vi "Build Monitor Cluster.vi"(8 "error in":errorcluster, 11 "custom device ref in":T4=18446744073709551615 format="%.0x") -> (0 "error out":errorcluster, 2 "Monitor cluster out":T1={"channel #"=0, "channel handle"=0, "InstrumentHandle_board"=0, "InstrumentHandle_port"=0, "Queue ID"=0, "channel settings"={"Monitor Settings"={"DefaultCronoMode"=0, "GlbMonBufferSizeIn"=0, "CaptureMode"=0, "MaxFileSize MB (1)"=1, "Strobe"=0, "TriggerPosition"=0}, "Rx Board"=0, "Rx Port"=0}, "File Reference"=refnum, "Monitor Log Directory"=""} {"channel settings"."Monitor Settings"."Strobe" items=["FDX_MON_STROBE_DIS", "FDX_MON_STROBE_STOP", "FDX_MON_STROBE_START"]; "channel settings"."Monitor Settings"."CaptureMode" items=["FDX_MON_SINGLE ", "FDX_MON_CONTINUOUS", "FDX_MON_SELECTIVE", "FDX_MON_RECORDING", "FDX_MON_REROS", "FDX_MON_HMU"]; "channel settings"."Monitor Settings"."DefaultCronoMode" items=["FDX_RX_DEFAULT_ENA_CNT", "FDX_RX_DEFAULT_MON_ENA_ALL", "FDX_RX_DEFAULT_MON_ENA_GOOD"]}, 3 "custom device ref out":T4 format="%.0x")   [LabVIEW 2020, in "afdx_custom_device Scripting.lvlib"]
uses:
  afdx_custom_device Scripting.lvlib
  <vilib>/NI VeriStand/Custom Device API/Custom Device Item Ref.ctl
  Engine/Implementation/Monitor Execution Unit/hardware_channels_rx.ctl
  Engine/Implementation/Monitor Execution Unit/channel_settings_rx.ctl
  AIM LabVIEW src/src/_controls/session_monitor_config.ctl
  Constants.vi
  <vilib>/NI VeriStand/Custom Device API/Get Item Property (U32).vi
  <vilib>/NI VeriStand/Custom Device API/Custom Device API.lvlib
  AIM LabVIEW src/src/AIM664LV.lvlib
  Engine/Implementation/Monitor Execution Unit/Monitor Execution Unit.lvclass
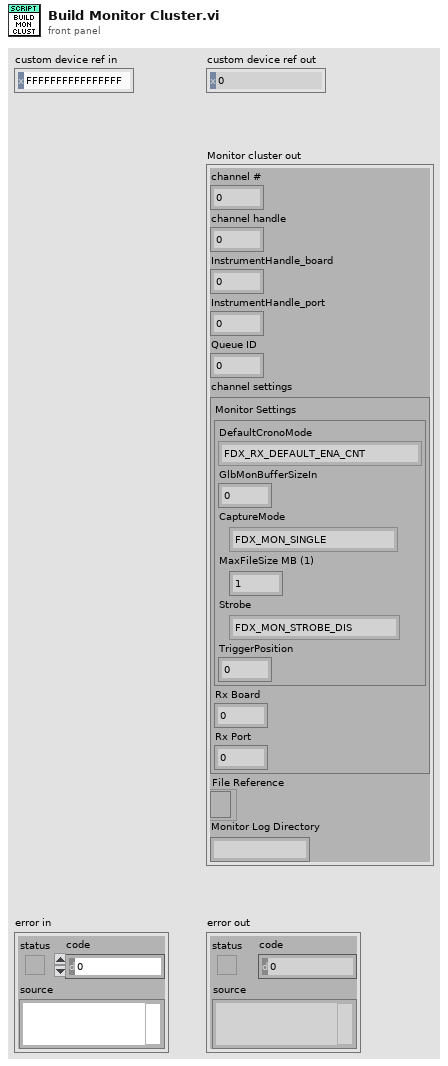
[diagram p1: front panel]
types:
  T1 = typedef "afdx_custom_device Engine.lvlib/Implementation.lvlib/Monitor Execution Unit.lvclass/hardware_channels_rx.ctl" = cluster{"channel #":u16, "channel handle":u64, "InstrumentHandle_board":u32, "InstrumentHandle_port":u32, "Queue ID":u32, "channel settings":T2, "File Reference":refnum<file>, "Monitor Log Directory":string}
  T2 = typedef "afdx_custom_device Engine.lvlib/Implementation.lvlib/Monitor Execution Unit.lvclass/channel_settings_rx.ctl" = cluster{"Monitor Settings":T3, "Rx Board":u32, "Rx Port":u32}
  T3 = typedef "AIM664LV.lvlib/session_monitor_config.ctl" = cluster{"DefaultCronoMode":u32, "GlbMonBufferSizeIn":u32, "CaptureMode":u32, "MaxFileSize MB (1)":u32, "Strobe":u32, "TriggerPosition":u32}
  T4 = typedef "Custom Device API.lvlib/Custom Device Item Ref.ctl" = u64
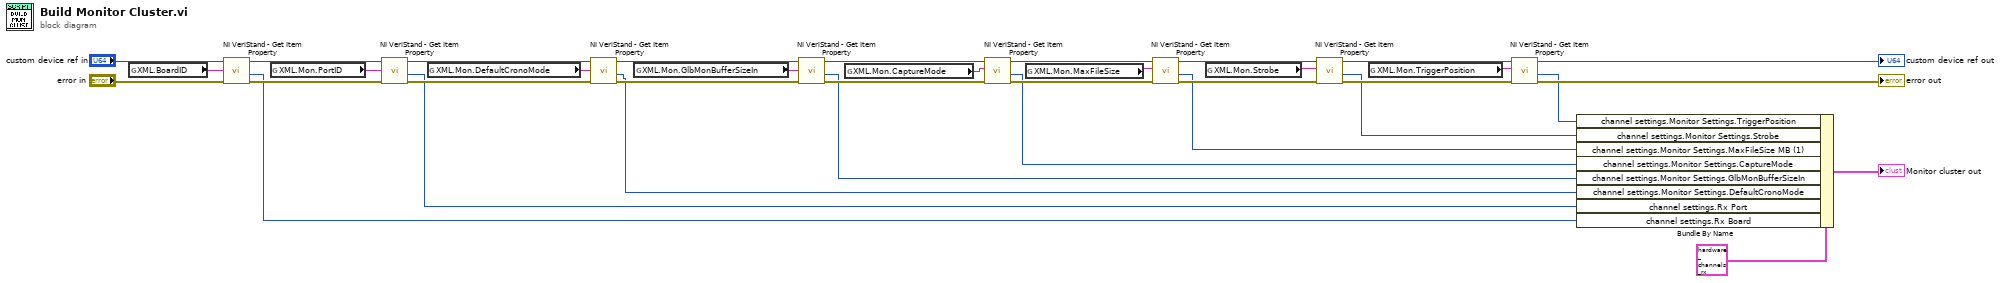
[diagram p0: block diagram]
diagram:
  n1 = global read "Constants.vi" "XML.BoardID"() -> (w1:string)
  n2 = call-poly <vilib>:"NI VeriStand - Get Item Property.vi"("error in (no error)"="error in", "Property Name"=w1, "Item Ref in"="custom device ref in") -> ("error out"=w3:errorcluster, "Value"=w2:u32, "Item Ref out"=w5:T4)  [unwired: 5 in, 1 out]
  n3 = global read "Constants.vi" "XML.Mon.PortID"() -> (w6:string)
  n4 = call-poly <vilib>:"NI VeriStand - Get Item Property.vi"("error in (no error)"=w3, "Property Name"=w6, "Item Ref in"=w5) -> ("error out"=w17:errorcluster, "Value"=w7:u32, "Item Ref out"=w18:T4)  [unwired: 5 in, 1 out]
  n5 = global read "Constants.vi" "XML.Mon.DefaultCronoMode"() -> (w8:string)
  n6 = call-poly <vilib>:"NI VeriStand - Get Item Property.vi"("error in (no error)"=w17, "Property Name"=w8, "Item Ref in"=w18) -> ("error out"=w16:errorcluster, "Value"=w9:u32, "Item Ref out"=w21:T4)  [unwired: 5 in, 1 out]
  n7 = global read "Constants.vi" "XML.Mon.GlbMonBufferSizeIn"() -> (w10:string)
  n8 = call-poly <vilib>:"NI VeriStand - Get Item Property.vi"("error in (no error)"=w16, "Property Name"=w10, "Item Ref in"=w21) -> ("error out"=w15:errorcluster, "Value"=w11:u32, "Item Ref out"=w19:T4)  [unwired: 5 in, 1 out]
  n9 = global read "Constants.vi" "XML.Mon.CaptureMode"() -> (w12:string)
  n10 = call-poly <vilib>:"NI VeriStand - Get Item Property.vi"("error in (no error)"=w15, "Property Name"=w12, "Item Ref in"=w19) -> ("error out"=w14:errorcluster, "Value"=w13:u32, "Item Ref out"=w20:T4)  [unwired: 5 in, 1 out]
  n11 = global read "Constants.vi" "XML.Mon.MaxFileSize"() -> (w29:string)
  n12 = call-poly <vilib>:"NI VeriStand - Get Item Property.vi"("error in (no error)"=w14, "Property Name"=w29, "Item Ref in"=w20) -> ("error out"=w31:errorcluster, "Value"=w26:u32, "Item Ref out"=w35:T4)  [unwired: 5 in, 1 out]
  n13 = global read "Constants.vi" "XML.Mon.Strobe"() -> (w28:string)
  n14 = call-poly <vilib>:"NI VeriStand - Get Item Property.vi"("error in (no error)"=w31, "Property Name"=w28, "Item Ref in"=w35) -> ("error out"=w30:errorcluster, "Value"=w24:u32, "Item Ref out"=w34:T4)  [unwired: 5 in, 1 out]
  n15 = global read "Constants.vi" "XML.Mon.TriggerPosition"() -> (w27:string)
  n16 = call-poly <vilib>:"NI VeriStand - Get Item Property.vi"("error in (no error)"=w30, "Property Name"=w27, "Item Ref in"=w34) -> ("error out"=→"error out":errorcluster, "Value"=w25:u32, "Item Ref out"=→"custom device ref out":T4)  [unwired: 5 in, 1 out]
  n17 = Bundle By Name(cluster=T1 {"channel #"=0, "channel handle"=0, "InstrumentHandle_board"=0, "InstrumentHandle_port"=0, "Queue ID"=0, "channel settings"={"Monitor Settings"={"DefaultCronoMode"=1, "GlbMonBufferSizeIn"=0, "CaptureMode"=0, "MaxFileSize MB (1)"=1, "Strobe"=0, "TriggerPosition"=0}, "Rx Board"=0, "Rx Port"=1}, "File Reference"=refnum, "Monitor Log Directory"="/home/"} ("RX Parameters"), "channel settings.Monitor Settings.TriggerPosition"=w25, "channel settings.Monitor Settings.Strobe"=w24, "channel settings.Monitor Settings.MaxFileSize MB (1)"=w26, "channel settings.Monitor Settings.CaptureMode"=w13, "channel settings.Monitor Settings.GlbMonBufferSizeIn"=w11, "channel settings.Monitor Settings.DefaultCronoMode"=w9, "channel settings.Rx Port"=w7, "channel settings.Rx Board"=w2) -> (→"Monitor cluster out":T1)
